vi "svfa_Average Spectrum (complex) (1 Ch).vi"(0 "spectrum":cluster{"f0":dbl, "df":dbl, "spectrum":cdb[]} {"spectrum" format="%.2p"; "df" format="%.2p"; "f0" format="%.2p"}, 1 "processing control":T1(ring), 7 "averaging parameters":T2={"averaging mode"=enum."No averaging", "weighting mode"=enum."Linear", "number of averages"=10, "linear mode"=enum."Auto restart"}, 11 "error in (no error)":errorcluster) -> (4 "spectrum":cluster{"f0":dbl, "df":dbl, "spectrum":cdb[]} {"spectrum" format="%.2p"; "df" format="%.2p"; "f0" format="%.2p"}, 8 "new spectrum ready":bool, 10 "averaging done":bool, 14 "averages completed":dbl, 15 "error out":errorcluster)   [LabVIEW 2017]
uses:
  <vilib>/addons/_NISVFA/_Shared subVIs/Spectrum Averaging/svfa_Reset Averaging State Info.vi
  <vilib>/addons/_NISVFA/_Shared subVIs/Spectrum Averaging/svfa_Average Array with Avg Checks (complex) No State.vi
  <vilib>/addons/_NISVFA/_Shared subVIs/Spectrum Averaging/svfa_Average Array (complex) No State.vi
  <vilib>/addons/_NISVFA/_Shared subVIs/Spectrum Averaging/svfa_No Average Array (complex).vi
  <vilib>/addons/_NISVFA/_Shared subVIs/Spectrum Averaging/svfa_Average Array (complex).vi
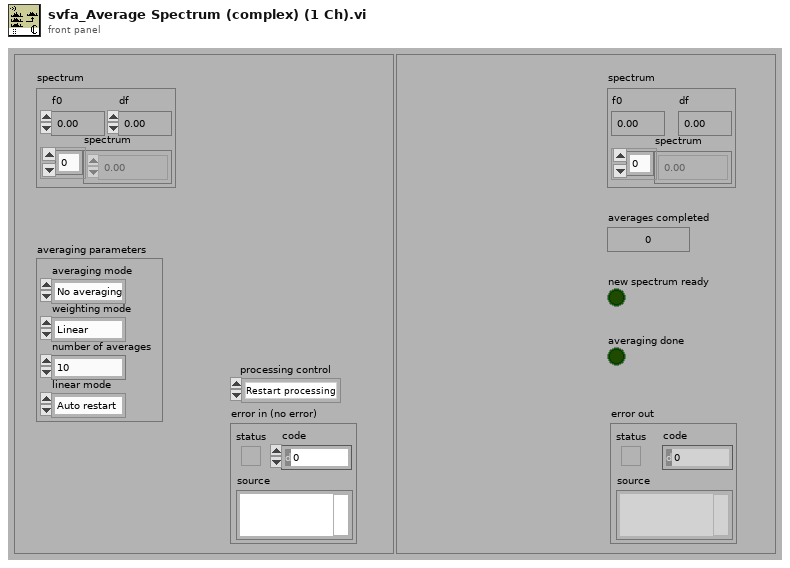
[diagram p1: front panel]
types:
  T1 = enum16{"Restart processing", "Continue processing", "Skip processing"}
  T2 = cluster{"averaging mode":enum16{"No averaging", "Vector averaging", "RMS averaging", "Peak hold"}, "weighting mode":enum16{"Linear", "Exponential"}, "number of averages":u32, "linear mode":enum16{"One shot", "Auto restart"}}
  T3 = cluster{"complex FFT":cdb[], "real FFT":dbl[], "f0":dbl, "df":dbl, "averages completed":dbl, "averaging parameters":cluster{"averaging mode":enum16{"No averaging", "Vector averaging", "RMS averaging", "Peak hold"}, "weighting mode":enum16{"Linear", "Exponential"}, "number of averages":u32, "linear mode":enum16{"One shot", "Auto restart"}}}
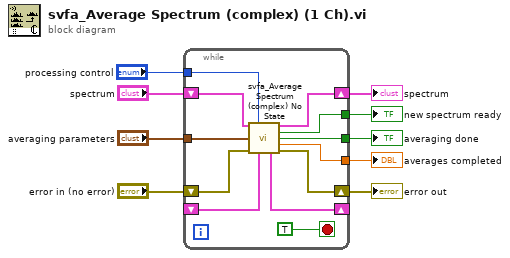
[diagram p0: block diagram]
diagram:
  n1 = while {
    tunnel: "processing control" -> [w10]
    tunnel: [w15] -> w2
    tunnel: [w16] -> w3
    tunnel: [w14] -> w5
    shift-left: _ -> [w18]
    shift-right: [w19] -> _
    tunnel: "averaging parameters" -> [w13]
    shift-right: [w17] -> w6
    shift-left: "spectrum" -> [w20]
    shift-right: [w11] -> w4
    shift-left: "error in (no error)" -> [w12]
    stop <- TRUE stop-if-true
    n2 = call <vilib>:"svfa_Average Spectrum (complex) No State.vi"("spectrum"=w20, "processing control"=w10, "averaging parameters"=w13, "error in (no error)"=w12, "averaging state info in"=w18) -> ("average spectrum"=w17:cluster{"f0":dbl, "df":dbl, "spectrum":cdb[]}, "new spectrum ready"=w14:bool, "averaging done"=w15:bool, "averages completed"=w16:dbl, "averaging state info out"=w19:T3, "error out"=w11:errorcluster)  [unwired: 5 in]
  }
  "averages completed" <- w3
  "spectrum" <- w6
  "averaging done" <- w2
  "new spectrum ready" <- w5
  "error out" <- w4
